vi "SSC DCPower Query In Compliance.vi"(0 "DCPower SSC in":T1[](array[typedef]), 11 "error in":errorcluster) -> (4 "DCPower SSC out":T1[](array[typedef]), 6 "In Compliance?":bool[](array[boolean]), 15 "error out":errorcluster)   [LabVIEW 2020]
doc: "Queries the specified output channels to determine if they is operating at the compliance limits."
uses:
  SSC DCPower.ctl
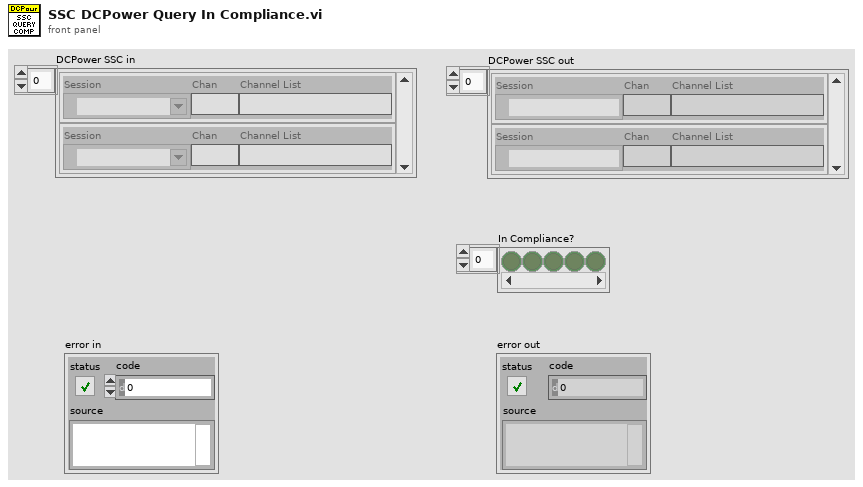
[diagram p1: front panel]
types:
  T1 = typedef "SSC DCPower.ctl" = cluster{"Session":refnum<k15>, "Chan":string, "Channel List":string}
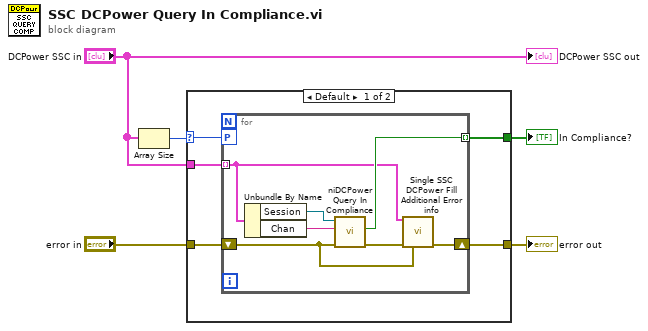
[diagram p0: block diagram]
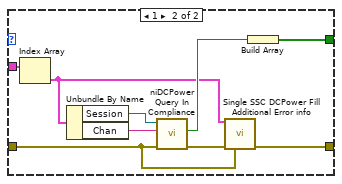
[diagram p2: hidden frame]
diagram:
  n1 = Array Size(array="DCPower SSC in") -> (size(s)=w2:i32)
  n2 = case shown="Default" w2 {
    selector: w2 -> [w7 _]
    tunnel: [w10 w26] -> w5
    tunnel: [w9 w18] -> w4
    tunnel: "error in" -> [w8 w24]
    tunnel: "DCPower SSC in" -> [w6 w23]
    frame Default {
      n3 = for {
        tunnel: w6 -> [w11] mode=indexing
        tunnel: [w16] -> w9 mode=indexing
        workers-P: w7 -> [_]
        shift-right: [w13] -> w10
        shift-left: w8 -> [w12]
        n4 = Unbundle By Name(w11) -> ("Session"=w15:refnum<k15>, "Chan"=w14:string)
        n5 = call <instrlib>:"niDCPower Query In Compliance.vi"("error in (no error)"=w12, "channel name"=w14, "instrument handle"=w15) -> ("error out"=w17:errorcluster, "in compliance?"=w16:bool)  [unwired: 6 in, 1 out]
        n6 = call "Single SSC DCPower Fill Additional Error info.vi"("DCPower SSC in"=w11, "error in"=w17, "previous error in"=w12) -> ("error out"=w13:errorcluster)  [unwired: 12 in]
      }
    }
    frame 1 {
      n7 = Index Array(array=w23) -> (element=w19:T1)  [unwired: 1 in]
      n8 = Unbundle By Name(w19) -> ("Session"=w21:refnum<k15>, "Chan"=w20:string)
      n9 = call <instrlib>:"niDCPower Query In Compliance.vi"("error in (no error)"=w24, "channel name"=w20, "instrument handle"=w21) -> ("error out"=w22:errorcluster, "in compliance?"=w25:bool)  [unwired: 6 in, 1 out]
      n10 = call "Single SSC DCPower Fill Additional Error info.vi"("DCPower SSC in"=w19, "error in"=w22, "previous error in"=w24) -> ("error out"=w26:errorcluster)  [unwired: 12 in]
      n11 = Build Array(w25) -> (w18:bool[])
    }
  }
  "error out" <- w5
  "In Compliance?" <- w4
  "DCPower SSC out" <- "DCPower SSC in"
